vi "Waveguide Model.vi"(2 "Vs (V)":dbl, 3 "Vsg (V)":dbl) -> (0 "I[Vsg] (A)":dbl, 1 "G[Vsg] (e2/h)":dbl)   [LabVIEW 2019, in "Instrument.DAQ.lvclass"]
uses:
  Instrument.DAQ.lvclass
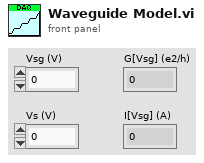
[diagram p1: front panel]
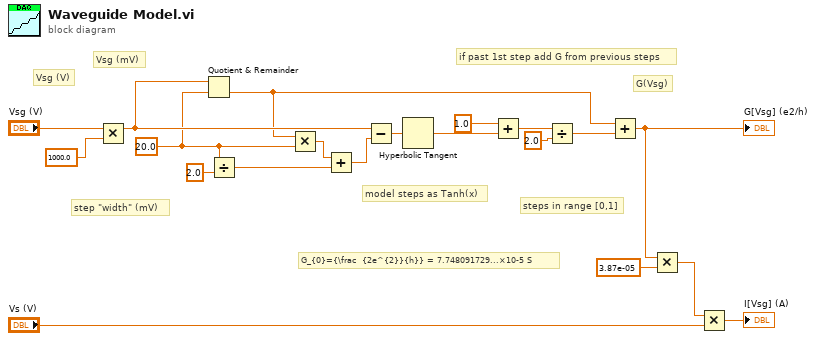
[diagram p0: block diagram]
diagram:
  w12 = 20.0 ("y")
  # "G_{0}={\\frac  {2e^{2}}{h}} = 7.748091729...×10-5 S"
  # "Vsg (mV)"
  # "if past 1st step add G from previous steps"
  # "steps in range [0,1]"
  # "model steps as Tanh(x)"
  # "step \"width\" (mV)"
  # "G(Vsg)"
  # "Vsg (V)"
  n1 = Multiply(x="Vsg (V)", y=1000.0) -> (x*y=w18:dbl)
  n2 = Quotient & Remainder(x=w18, y=w12) -> (floor(x/y)=w13:dbl)  [unwired: 1 out]
  n3 = Divide(x=w12, y=2.0) -> (x/y=w10:dbl)
  n4 = Multiply(x=w13, y=w12) -> (x*y=w7:dbl)
  n5 = Add(x=w7, y=w10) -> (x+y=w8:dbl)
  n6 = Subtract(x=w18, y=w8) -> (x-y=w2:dbl)
  n7 = Hyperbolic Tangent(1:w2) -> (0:w6:dbl)
  n8 = Add(x=1.0, y=w6) -> (x+y=w4:dbl)
  n9 = Divide(x=w4, y=2.0) -> (x/y=w1:dbl)
  n10 = Add(x=w13, y=w1) -> (x+y=w16:dbl)
  "G[Vsg] (e2/h)" <- w16
  n11 = Multiply(x=w16, y=3.87e-05) -> (x*y=w20:dbl)
  n12 = Multiply(x=w20, y="Vs (V)") -> (x*y=→"I[Vsg] (A)":dbl)
